vi "PC Keyboard Control.vi"(3 "Rudder":u8(knob)=7, 4 "Prop":u8(slide)=7 scale=0.0..14.0, 5 "IR Servo":u8(knob)=7 scale=0.0..14.0) -> ()   [LabVIEW 2012]
uses:
  <vilib>/Utility/inputDevices.llb/closeKeyboard.vi
  <vilib>/Utility/inputDevices.llb/keyboardAcquire.vi
panel:
  out "Key Output":i32
  out "Vertical Output":i32
  out "Horizontal Output":i32
  out "Key code":i32[](array[numeric])
  out "keys pressed":T1(array[ring])
  out "string":string
  out "error in 2":errorcluster
  out "return count":u32
  out "String Received":string
  out "String":string="$B^"
  in  "error in":errorcluster
  in  "VISA resource name":refnum<visa-resource-name>="COM10"
  out "Heartbeat":bool
  out "Soft Stop\nEngaged":bool
  out "Base\nStation?":bool
  out "Boat?":bool
  in  "SOFT E-STOP":bool
  in  "HARD E-STOP":bool
  in  "# 5":u8 max=5 step=1
  in  "# 4":u8 max=5 step=1
  in  "# 3":u8 max=5 step=1
  in  "# 2":u8 max=5 step=1
  in  "# 1":u8 max=5 step=1
  in  "# 0":u8=1 max=5 step=1
  out "IR Time":dbl
  out "IR Dist":dbl
  # "Behavior\nWeights"
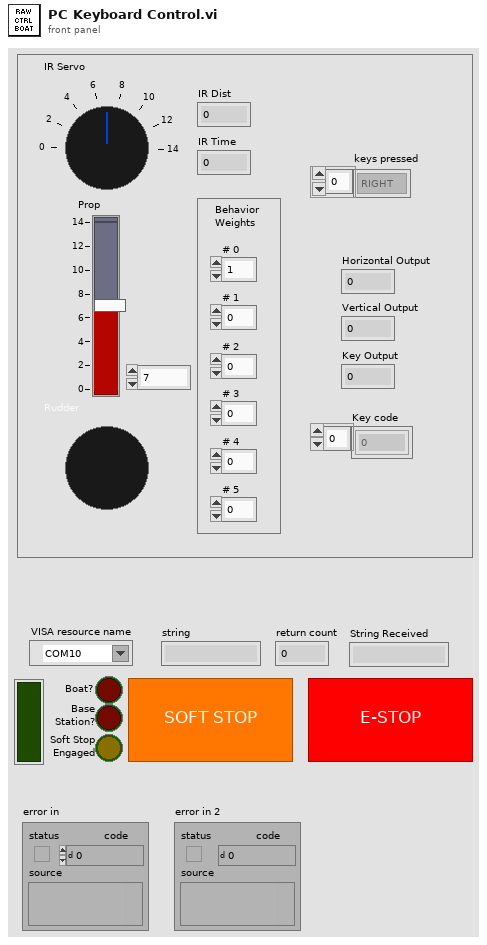
[diagram p1: front panel]
types:
  T1 = enum16{"0", "1", "2", "3", "4", "5", "6", "7", "8", "9", "A", "B", "C", "D", "E", "F", "G", "H", "I", "J", "K", "L", "M", "N", "O", "P", "Q", "R", "S", "T", "U", "V", "W", "X", "Y", "Z", "F1", "F2", "F3", "F4", "F5", "F6", "F7", "F8", "F9", "F10", "F11", "F12", "F13", "F14", "F15", "ADD", "BACK", "BACKSLASH", "CAPITAL", "COMMA", "DECIMAL", "DELETE", "DIVIDE", "DOWN", "END", "EQUALS", "ESCAPE", "GRAVE (`)", "HOME", "INSERT", "LBRACKET", "LCONTROL", "LEFT", "L ALT", "LSHIFT", "LWIN", "MINUS", "MULTIPLY", "NEXT", "NUMLOCK", "NUMPAD_0", "NUMPAD_1", "NUMPAD_2", "NUMPAD_3", "NUMPAD_4", "NUMPAD_5", "NUMPAD_6", "NUMPAD_7", "NUMPAD_8", "NUMPAD_9", "PAUSE", "PERIOD", "PRIOR (PG UP)", "RBRACKET", "RCONTROL", "RETURN", "RIGHT", "R ALT", "RSHIFT", "RWIN", "SCROLL", "SEMICOLON", "SLASH", "SPACE", "SUBTRACT", "TAB", "UP", "ENTER (num pad)", "' (quote)"}[]
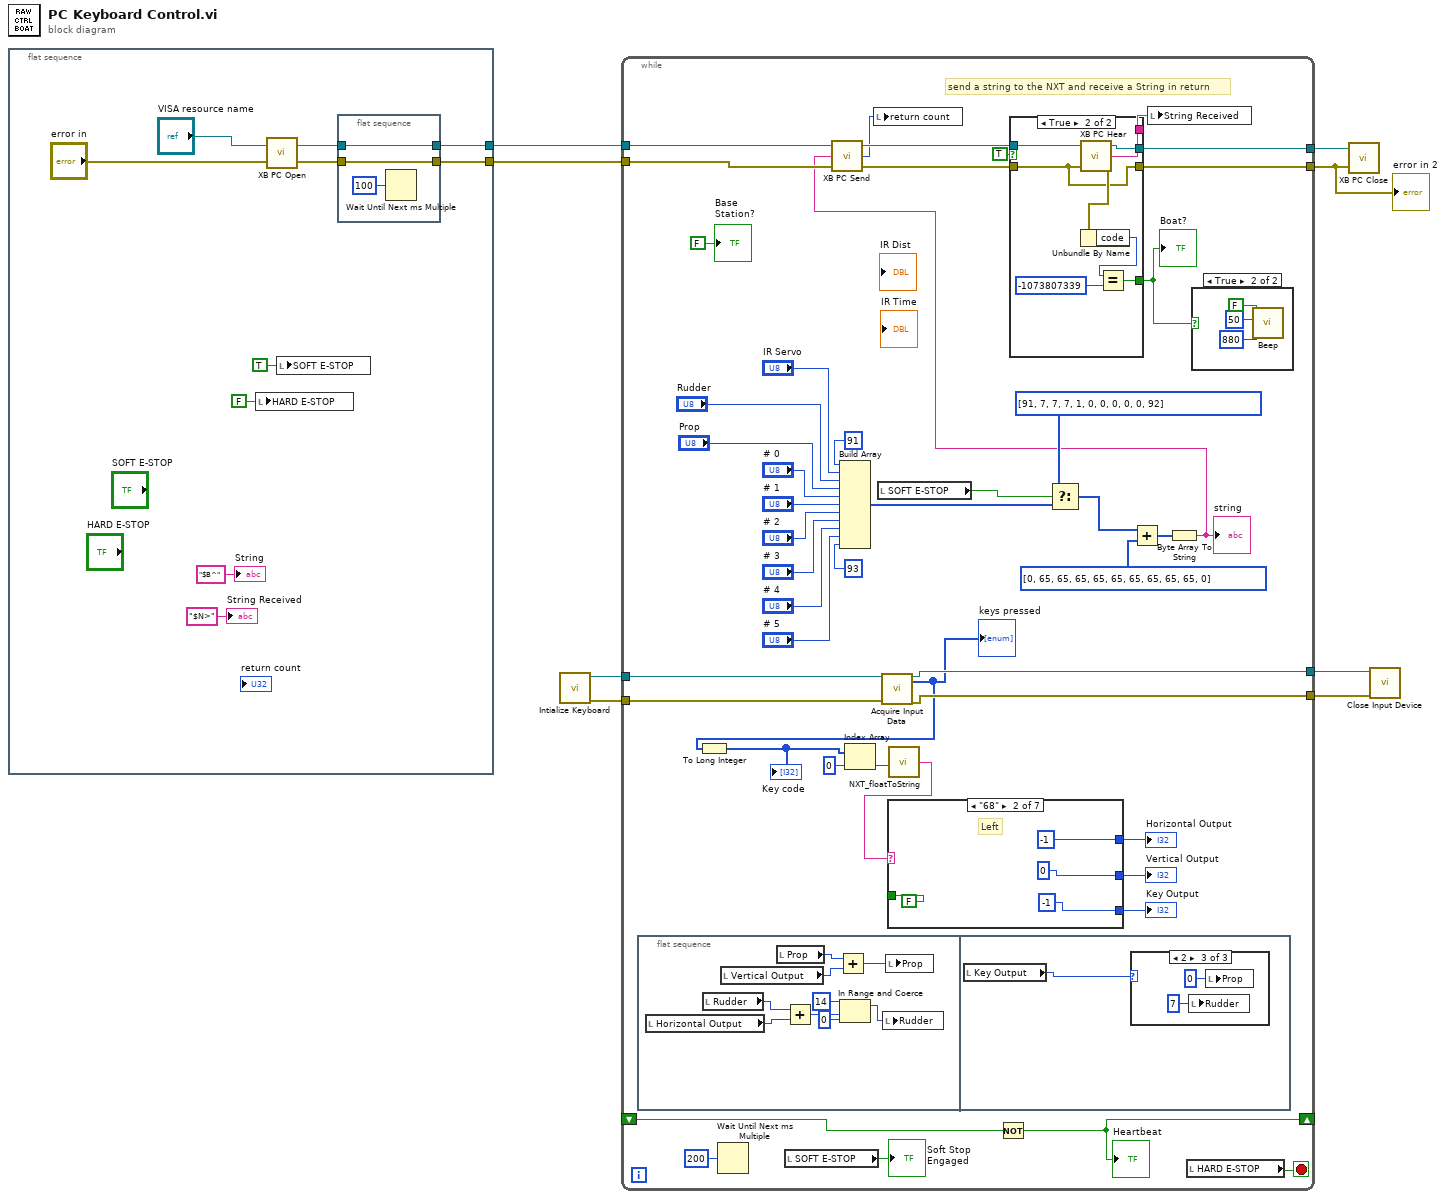
[diagram p0: block diagram]
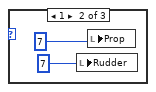
[diagram p3: hidden frame]
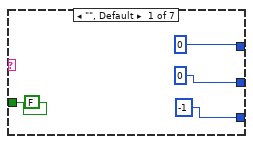
[diagram p4: hidden frame]
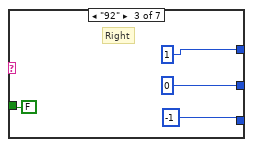
[diagram p5: hidden frame]
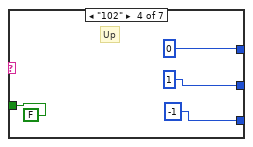
[diagram p6: hidden frame]
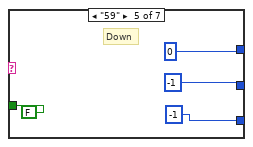
[diagram p7: hidden frame]
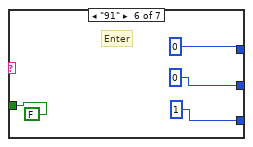
[diagram p8: hidden frame]
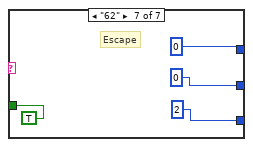
[diagram p9: hidden frame]
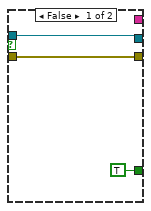
[diagram p11: hidden frame]
diagram:
  n1 = flat-sequence {
    tunnel: [w14] -> w8
    tunnel: [w13] -> w7
    frame #0 {
      n2 = local write "HARD E-STOP"(FALSE ("HARD E-STOP")) -> ()
      n3 = call "XB PC Open.vi"("error in (no error)"="error in", "VISA resource name"="VISA resource name") -> ("error out"=w17:errorcluster, "VISA resource name out"=w18:refnum<visa-resource-name>)
      n4 = local write "SOFT E-STOP"(TRUE ("SOFT E-STOP")) -> ()
      n5 = flat-sequence {
        tunnel: w18 -> [w19]
        tunnel: w17 -> [w20]
        tunnel: [w20] -> w13
        tunnel: [w19] -> w14
        frame #0 {
          n6 = Wait Until Next ms Multiple(millisecond multiple=u32 100) -> ()  [unwired: 1 out]
        }
      }
      "String" <- "$B^" ("String")
      "String Received" <- "$N>" ("String Received")
    }
  }
  n7 = call <vilib>:"Intialize Keyboard.vi"() -> ("error out"=w3:errorcluster, "device ID"=w4:refnum<k1>)  [unwired: 10 in]
  n8 = while {
    tunnel: w8 -> [w67]
    tunnel: w7 -> [w66]
    tunnel: [w65] -> w6
    tunnel: [w64] -> w5
    shift-right: [w48] -> _
    shift-left: _ -> [w47]
    tunnel: w4 -> [w33]
    tunnel: w3 -> [w32]
    tunnel: [w31] -> w2
    tunnel: [w30] -> w1
    stop <- w49 stop-if-true
    # "send a string to the NXT and receive a String in return"
    n9 = flat-sequence {
      frame #0 {
        n10 = local read "Horizontal Output"() -> (w72:i32)
        n11 = local read "Rudder"() -> (w73:u8)
        n12 = local read "Vertical Output"() -> (w75:i32)
        n13 = local read "Prop"() -> (w76:u8)
        n14 = Add(x=w73, y=w72) -> (x+y=w70:i32)
        n15 = Add(x=w76, y=w75) -> (x+y=w74:i32)
        n16 = In Range and Coerce(upper limit=14, x=w70, lower limit=0) -> (coerced(x)=w71:i32)  [unwired: 1 out]
        n17 = local write "Rudder"(w71) -> ()
        n18 = local write "Prop"(w74) -> ()
      }
      frame #1 {
        n19 = local read "Key Output"() -> (w77:i32)
        n20 = case shown="2" w77 {
          frame 0, Default {
          }
          frame 1 {
            n21 = local write "Rudder"(7) -> ()
            n22 = local write "Prop"(7) -> ()
          }
          frame 2 {
            n23 = local write "Rudder"(u8 7 ("Rudder")) -> ()
            n24 = local write "Prop"(u8 0 ("Prop")) -> ()
          }
        }
      }
    }
    n25 = Wait Until Next ms Multiple(millisecond multiple=u32 200) -> ()  [unwired: 1 out]
    n26 = local read "SOFT E-STOP"() -> (→"Soft Stop\nEngaged":bool)
    n27 = Build Array(u8 91 ("element"), "IR Servo", "Rudder", "Prop", "# 0", "# 1", "# 2", "# 3", "# 4", "# 5", u8 93 ("element")) -> (w56:u8[])
    n28 = local read "SOFT E-STOP"() -> (w55:bool)
    n29 = call-poly <vilib>:"Acquire Input Data.vi"("device ID"=w33, "error in (no error)"=w32) -> ("device ID"=w31:refnum<k1>, "keys pressed"=w23:T1, "error out"=w30:errorcluster)  [unwired: 15 in]
    "keys pressed" <- w23
    n30 = To Long Integer(number=w23) -> (32bit integer=w29:i32[])
    "Key code" <- w29
    n31 = Index Array(array=w29, index=0) -> (element=w27:i32)
    n32 = call <vilib>:"NXT_floatToString.vi"("number"=w27) -> ("string"=w22:string)
    n33 = case shown="\"68\"" w22 {
      tunnel: [FALSE FALSE FALSE FALSE FALSE FALSE TRUE] -> _
      tunnel: [0 -1 1 0 0 0 0] -> w26
      tunnel: [0 0 0 1 -1 0 0] -> w25
      tunnel: [-1 -1 -1 -1 -1 1 2] -> w24
      frame "", Default {
      }
      frame "68" {
        # "Left"
      }
      frame "92" {
        # "Right"
      }
      frame "102" {
        # "Up"
      }
      frame "59" {
        # "Down"
      }
      frame "91" {
        # "Enter"
      }
      frame "62" {
        # "Escape"
      }
    }
    "Horizontal Output" <- w26
    "Vertical Output" <- w25
    "Key Output" <- w24
    n34 = Not(x=w47) -> (.not. x?=w48:bool)
    "Heartbeat" <- w48
    n35 = Select(t=u8[] [91, 7, 7, 7, 1, 0, 0, 0, 0, 0, 92], s=w55, f=w56) -> (s? t:f=w44:u8[])
    n36 = Add(x=w44, y=u8[] [0, 65, 65, 65, 65, 65, 65, 65, 65, 65, 0]) -> (x+y=w43:u8[])
    n37 = Byte Array To String(unsigned byte array=w43) -> (string=w37:string)
    "string" <- w37
    n38 = call "XB PC Send.vi"("error in (no error)"=w66, "String"=w37, "VISA resource name"=w67) -> ("error out"=w54:errorcluster, "return count"=w50:u32, "VISA resource name out"=w53:refnum<visa-resource-name>)
    n39 = local write "return count"(w50) -> ()
    n40 = case shown="True" TRUE {
      tunnel: [w115 w123] -> w65
      tunnel: [w114 w116] -> w64
      tunnel: w54 -> [w114 w116]
      tunnel: w53 -> [w115 w122]
      tunnel: [_ w121] -> w51
      tunnel: [TRUE w117] -> w36
      frame False {
      }
      frame True {
        n41 = call "XB PC Hear.vi"("VISA resource name"=w122, "error in (no error)"=w116) -> ("VISA resource name out"=w123:refnum<visa-resource-name>, "String Received"=w121:string, "error out"=w120:errorcluster)
        n42 = Unbundle By Name(w120) -> ("code"=w119:i32)
        n43 = Equal?(x=w119, y=-1073807339) -> (x = y?=w117:bool)
      }
    }
    "Boat?" <- w36
    n44 = local write "String Received"(w51) -> ()
    n45 = local read "HARD E-STOP"() -> (w49:bool)
    n46 = case shown="True" w36 {
      frame False {
      }
      frame True {
        n47 = call <vilib>:"Beep.vi"("use system alert? (T)"=FALSE, "duration (msec)"=u32 50, "frequency (Hz)"=u32 880) -> ()  [unwired: 9 in]
      }
    }
    "Base\nStation?" <- FALSE ("Base\nStation?")
  }
  "error in 2" <- w5
  n48 = call "XB PC Close.vi"("error in (no error)"=w5, "VISA resource name"=w6) -> ()
  n49 = call-poly <vilib>:"Close Input Device.vi"("error in (no error)"=w1, "device ID"=w2) -> ()  [unwired: 8 in, 1 out]
